vi "FGV_config.vi"(7 "FGV states":T2, 8 "error in (no error)":errorcluster) -> (0 "error out":errorcluster, 3 "Settings":T1)   [LabVIEW 2020]
uses:
  FGVstates.ctl
  settings.ctl
  <vilib>/Utility/config.llb/Read Key (Path).vi
  <vilib>/Utility/config.llb/Read Key (I32).vi
  <vilib>/Utility/config.llb/NI_LVConfig.lvlib
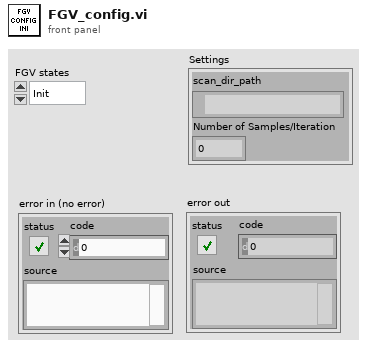
[diagram p1: front panel]
types:
  T1 = typedef "settings.ctl" = cluster{"scan_dir_path":path, "Number of Samples/Iteration":i32}
  T2 = typedef "FGVstates.ctl" = enum16{"Init", "Set", "Get", "De-Init"}
  T3 = typedef "NI_LVConfig.lvlib/Config Data RefNum.ctl" = refnum<k1>
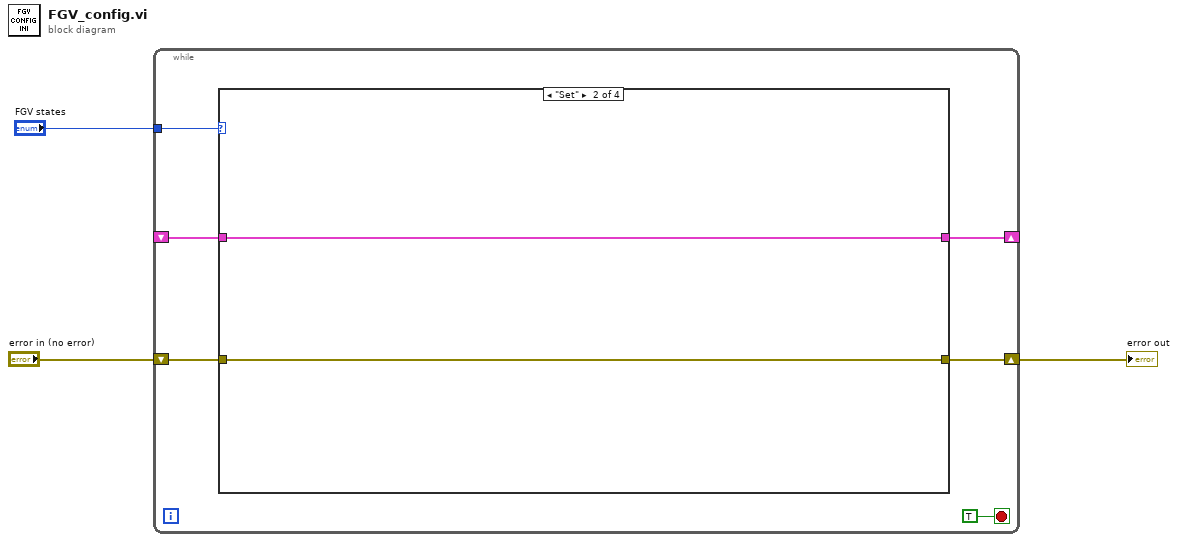
[diagram p0: block diagram]
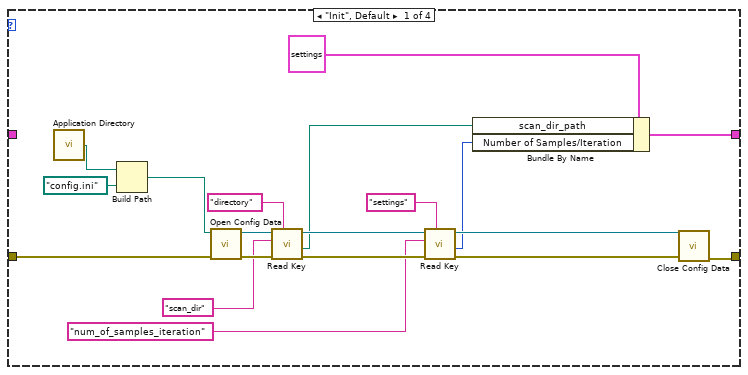
[diagram p2: hidden frame]
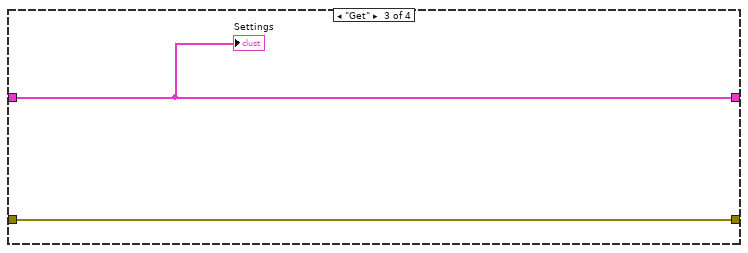
[diagram p3: hidden frame]
diagram:
  n1 = while {
    tunnel: "FGV states" -> [w8]
    shift-right: [w6] -> w1
    shift-left: "error in (no error)" -> [w7]
    shift-right: [w5] -> _
    shift-left: _ -> [w4]
    stop <- TRUE stop-if-true
    n2 = case shown="\"Set\"" w8 {
      tunnel: w7 -> [w28 w30 w32 w34]
      tunnel: [w20 w30 w32 w34] -> w6
      tunnel: [w10 w29 w31 w33] -> w5
      tunnel: w4 -> [_ w29 w31 w33]
      frame "Init", Default {
        n3 = call <vilib>:"Application Directory.vi"() -> ("Application Directory"=w25:path)
        n4 = Build Path(base path=w25, name or relative path=path "config.ini") -> (appended path=w23:path)
        n5 = call <vilib>:"Open Config Data.vi"("error in (no error)"=w28, "configuration file path"=w23) -> ("error out"=w27:errorcluster, "refnum"=w26:T3)  [unwired: 7 in, 1 out]
        n6 = call-poly <vilib>:"Read Key.vi"("section"="directory", "error in (no error)"=w27, "key"="scan_dir", "refnum"=w26) -> ("error out"=w18:errorcluster, "value"=w11:path, "refnum out"=w19:T3)  [unwired: 4 in, 1 out]
        n7 = call-poly <vilib>:"Read Key.vi"("section"="settings", "error in (no error)"=w18, "key"="num_of_samples_iteration", "refnum"=w19) -> ("error out"=w15:errorcluster, "value"=w12:i32, "refnum out"=w14:T3)  [unwired: 4 in, 1 out]
        n8 = Bundle By Name(cluster=T1 {"scan_dir_path"=path "D:/_LabVIEW/Projects/WavPlayer/Music", "Number of Samples/Iteration"=2500} ("Settings"), "scan_dir_path"=w11, "Number of Samples/Iteration"=w12) -> (w10:T1)
        n9 = call <vilib>:"Close Config Data.vi"("error in (no error)"=w15, "refnum"=w14) -> ("error out"=w20:errorcluster)  [unwired: 8 in, 1 out]
      }
      frame "Set" {
      }
      frame "Get" {
        "Settings" <- w31
      }
      frame "De-Init" {
      }
    }
  }
  "error out" <- w1
